vi "Add View.vi"(8 "error in (no error)":errorcluster, 10 "Debug Process":refnum<class "Debug View.lvclass">, 11 "Messages Composite View In":refnum<class "Messages Composite View.lvclass">) -> (0 "error out":errorcluster, 3 "Messages Composite View Out":refnum<class "Messages Composite View.lvclass">)   [LabVIEW 2020, in "Messages Composite View.lvclass"]
uses:
  Messages Composite View.lvclass
  Debug View/Debug View.lvclass
  Messages Composite View.lvclass/Messages Composite View.ctl
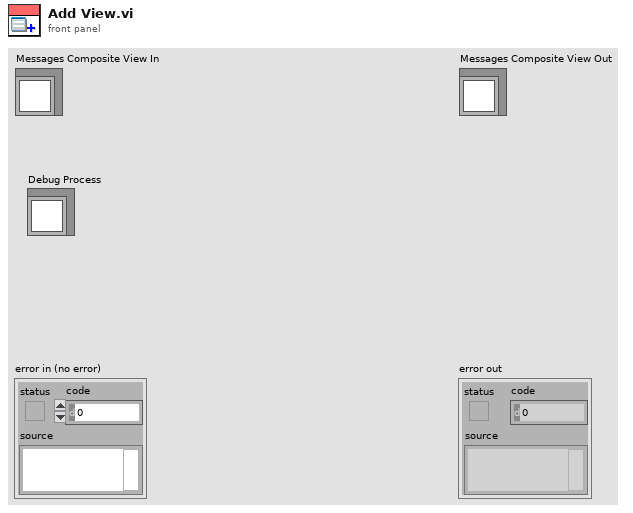
[diagram p1: front panel]
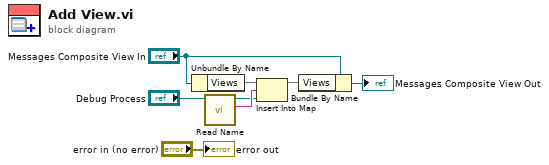
[diagram p0: block diagram]
diagram:
  n1 = Unbundle By Name("Messages Composite View In") -> ("Views"=w4:map{string, refnum<class "Debug View.lvclass">})
  n2 = call "Read Name.vi"("Process In"="Debug Process") -> ("Name"=w2:string, "Process Out"=w1:refnum<class "Debug View.lvclass">)  [unwired: 8 in, 1 out]
  n3 = Insert Into Map(map in=w4, key=w2, value=w1) -> (map out=w3:map{string, refnum<class "Debug View.lvclass">})  [unwired: 2 out]
  n4 = Bundle By Name(cluster="Messages Composite View In", "Views"=w3) -> (→"Messages Composite View Out":refnum<class "Messages Composite View.lvclass">)
  "error out" <- "error in (no error)"
